vi "View File.vi"(8 "error in":errorcluster, 11 "CSV in":refnum<class "CSV.lvclass">) -> (0 "error out":errorcluster, 3 "CSV out":refnum<class "CSV.lvclass">)   [LabVIEW 2020, in "Manejador archivo.lvlib" / "CSV.lvclass"]
uses:
  CSV.lvclass
  C:/GitClones/DQMH-LabVIEW-GYM/10 Mayo/04 DQMH USER/Libraries/Manejador archivo/Class Definitions/File/File.lvclass
  File/File.lvclass/File.ctl
  File/Read File Path.vi
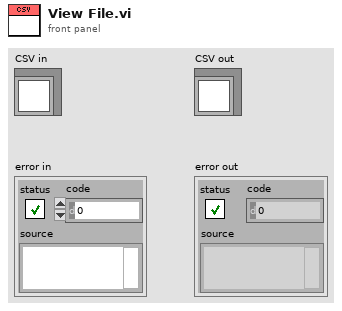
[diagram p1: front panel]
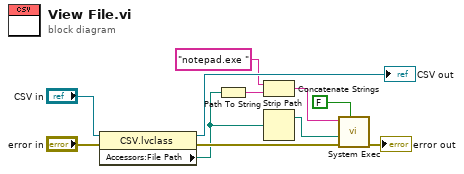
[diagram p0: block diagram]
diagram:
  n1 = property class="CSV.lvclass"(reference="CSV in", error in="error in") -> (reference out=→"CSV out":refnum<class "CSV.lvclass">, error out=w10:errorcluster, "Accessors:File Path"=w1:path)
  n2 = Path To String(path=w1) -> (string=w2:string)
  n3 = Concatenate Strings("notepad.exe " ("command line"), w2) -> (w3:string)
  n4 = Strip Path(path=w1) -> (stripped path=w4:path)  [unwired: 1 out]
  n5 = call <vilib>:"System Exec.vi"("wait until completion? (T)"=FALSE, "error in (no error)"=w10, "working directory"=w4, "command line"=w3) -> ("error out"=→"error out":errorcluster)  [unwired: 4 in, 3 out]
